vi "connection_count.vi"(8 "error in (no error)":errorcluster, 11 "TCP Socket Server in":refnum<class "TCP Socket Server.lvclass">) -> (0 "error out":errorcluster, 2 "connection count":i32, 3 "TCP Socket Server out":refnum<class "TCP Socket Server.lvclass">)   [LabVIEW 2019, in "TCP Socket Server.lvclass"]
uses:
  TCP Socket Server.lvclass
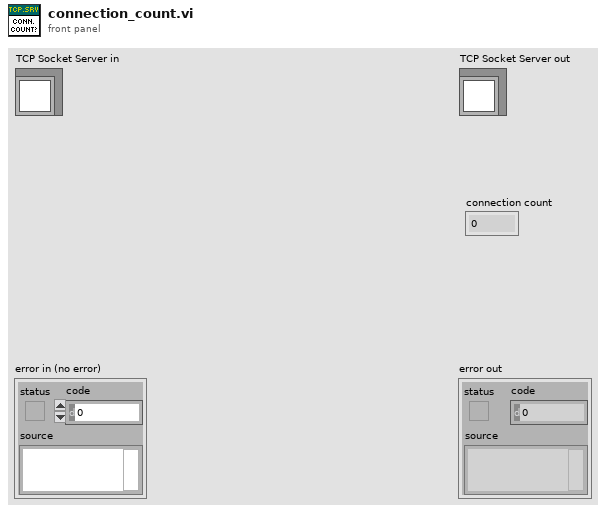
[diagram p1: front panel]
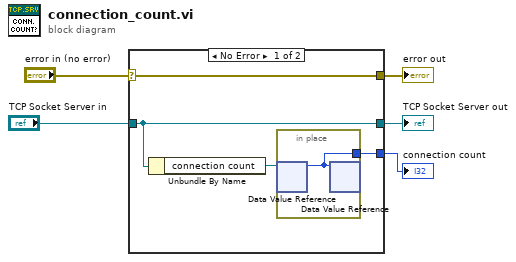
[diagram p0: block diagram]
diagram:
  n1 = case shown="No Error" "error in (no error)" {
    selector: "error in (no error)" -> [w9 w12]
    tunnel: [w9 w12] -> w4
    tunnel: [w8 w11] -> w2
    tunnel: "TCP Socket Server in" -> [w8 w11]
    tunnel: [w6 _] -> w1
    frame No Error {
      n2 = Unbundle By Name(w8) -> ("connection count"=w7:refnum<data-value>)
      n3 = in-place {
        in-place-border: [w10] -> w6
        n4 = in-place-dvr #1(w7) -> (w10:i32)  [unwired: 1 out]
        n5 = in-place-dvr #1(w10) -> ()  [unwired: 2 out]
      }
    }
    frame Error {
    }
  }
  "error out" <- w4
  "TCP Socket Server out" <- w2
  "connection count" <- w1
